vi "Lab5-Spectrum_Analyzer.vi"() -> ()   [LabVIEW 2016]
uses:
  <vilib>/Analysis/4window.llb/windowTd.ctl
  <vilib>/measure/madcrms.llb/Averaged DC-RMS for N Chan.vi
  <vilib>/measure/mascope.llb/Amplitude and Levels N chan.vi
  <vilib>/measure/maspectr.llb/FFT Power Spectrum and PSD for N Chan.vi
  <vilib>/measure/NI_MAPro.lvlib
  <vilib>/Analysis/NI_AALPro.lvlib
panel:
  out "RMS value waveforms":waveform(dbl)[](array[waveform])
  out "amplitude":dbl[](array[numeric]) format="%.2p"
  in  "averaging parameters":T1={"averaging mode"=enum."No averaging", "weighting mode"=enum."Exponential", "number of averages"=10} {"number of averages" min=1}
  in  "window":T2=1 items=["Rectangle"=0, "Hanning"=1, "Hamming"=2, "Blackman-Harris"=3, "Exact Blackman"=4, "Blackman"=5, "Flat Top"=6, "4 Term B-Harris "=7, "7 Term B-Harris"=8, "Low Sidelobe"=9, "Blackman Nuttall"=11, "Triangle"=30, "Bartlett-Hanning"=31, "Bohman"=32, "Parzen"=33, "Welch"=34, "Kaiser"=60, "Dolph-Chebyshev"=61, "Gaussian"=62]
  in  "dB On (F)":bool
  in  "number of samples":i32=100
  in  "rate":dbl=1000.0
  out "Waveform Graph":dynamicdata(graph)
  in  "stop":bool
  out "Power Spectrum":cluster{"f0":dbl, "df":dbl, "magnitude":dbl[]}[](graph)
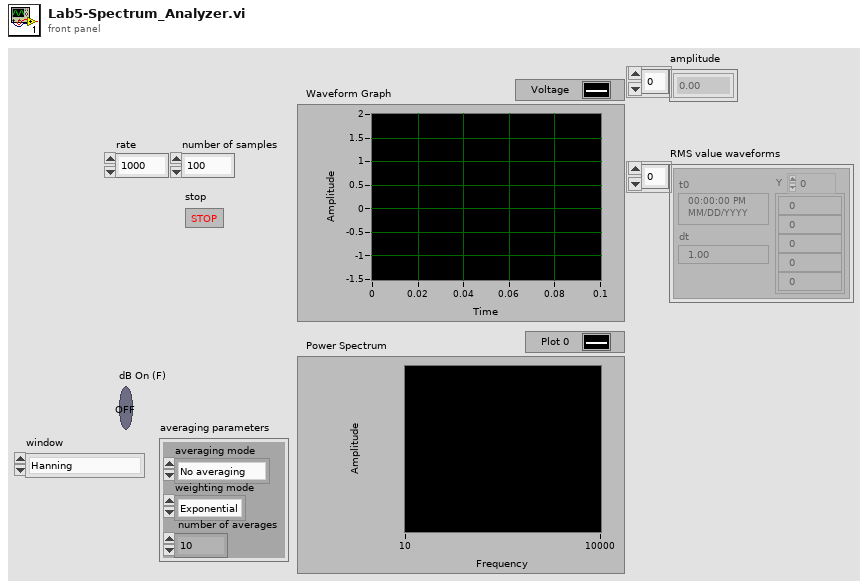
[diagram p1: front panel]
types:
  T1 = cluster{"averaging mode":enum16{"No averaging", "Vector averaging", "RMS averaging", "Peak hold"}, "weighting mode":enum16{"Linear", "Exponential"}, "number of averages":u32}
  T2 = typedef "NI_AALPro.lvlib/windowTd.ctl" = u32
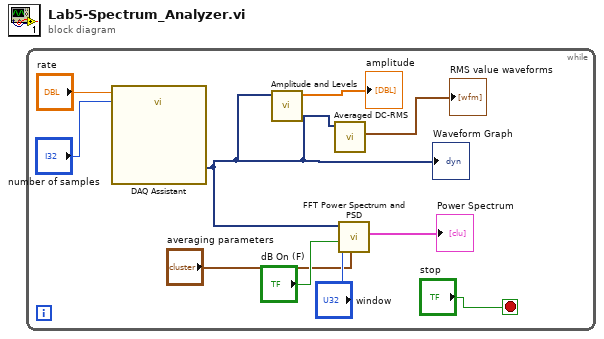
[diagram p0: block diagram]
diagram:
  n1 = while {
    stop <- "stop" stop-if-true
    n2 = call "DAQ Assistant"("rate"="rate", "number of samples"="number of samples") -> ("data"=w2:dynamicdata)  [unwired: 14 in, 3 out]
    "Waveform Graph" <- w2
    n3 = call-poly <vilib>:"Amplitude and Levels.vi"("signal(s) in"=w2) -> ("amplitude"=→"amplitude":dbl[])  [unwired: 7 in, 3 out]
    n4 = call-poly <vilib>:"Averaged DC-RMS.vi"("signals in"=w2) -> ("RMS value waveforms"=→"RMS value waveforms":waveform(dbl)[])  [unwired: 6 in, 4 out]
    n5 = call-poly <vilib>:"FFT Power Spectrum and PSD.vi"("averaging parameters"="averaging parameters", "dB On (F)"="dB On (F)", "window"="window", "time signals"=w2) -> ("Power Spectrum / PSD"=→"Power Spectrum":cluster{"f0":dbl, "df":dbl, "magnitude":dbl[]}[])  [unwired: 4 in, 3 out]
  }
